vi "Read configuration.vi"(8 "error in":errorcluster, 11 "PID Module 2 editor node in":refnum<class "PID Module 2 editor node.lvclass">) -> (0 "error out":errorcluster, 2 "configuration":refnum<class "NISE_CEF_serializable configuration.lvclass">, 3 "PID Module 2 editor node out":refnum<class "PID Module 2 editor node.lvclass">)   [LabVIEW 2015, in "PID Module 2 editor node.lvclass"]
uses:
  PID Module 2 editor node.lvclass
  <vilib>/NI/Configuration Framework/serializable configuration/NISE_CEF_serializable configuration.lvclass
  PID Module 2 editor node.lvclass/PID Module 2 editor node.ctl
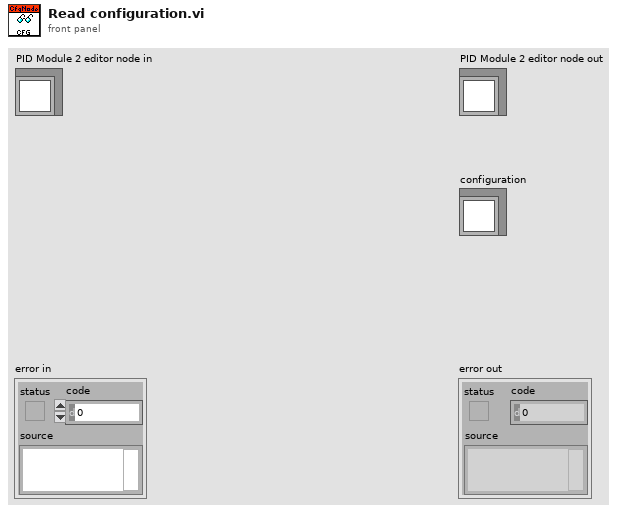
[diagram p1: front panel]
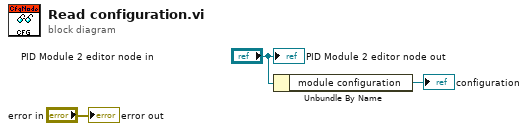
[diagram p0: block diagram]
diagram:
  n1 = Unbundle By Name("PID Module 2 editor node in") -> ("module configuration"=→"configuration":refnum<class "PID Module 2 configuration.lvclass">)
  "error out" <- "error in"
  "PID Module 2 editor node out" <- "PID Module 2 editor node in"
